vi "Open Item.vi"(8 "error in (no error)":errorcluster, 10 "Item name":string, 11 "Measure Object in":refnum<class "da Base.lvclass">) -> (0 "error out":errorcluster, 3 "Measure Object out":refnum<class "da Base.lvclass">)   [LabVIEW 2016, in "da Base.lvclass"]
uses:
  da Base.lvclass
  C:/Program Files/National Instruments/LabVIEW 2016/vi.lib/ActorFramework/Actor/Actor.lvclass
  <vilib>/ActorFramework/Actor/Actor.lvclass/Actor.ctl
  Da Base Messages/Open Item Msg/Open Item Msg.lvclass/Open Item Msg.ctl
  <vilib>/ActorFramework/Message Enqueuer/Message Enqueuer.lvclass/Message Enqueuer.ctl
  <vilib>/ActorFramework/Message Enqueuer/Enqueue.vi
  Da Base Messages/Open Item Msg/Open Item Msg.lvclass
  C:/Program Files/National Instruments/LabVIEW 2016/vi.lib/ActorFramework/Message/Message.lvclass
  Da Base Messages/Open Front Panel Msg/Open Front Panel Msg.lvclass
  <vilib>/ActorFramework/Message Priority Queue/Priority Enqueue.vi
  <vilib>/ActorFramework/Message Enqueuer/Message Enqueuer.lvclass
  <vilib>/ActorFramework/Actor/Actor.lvclass
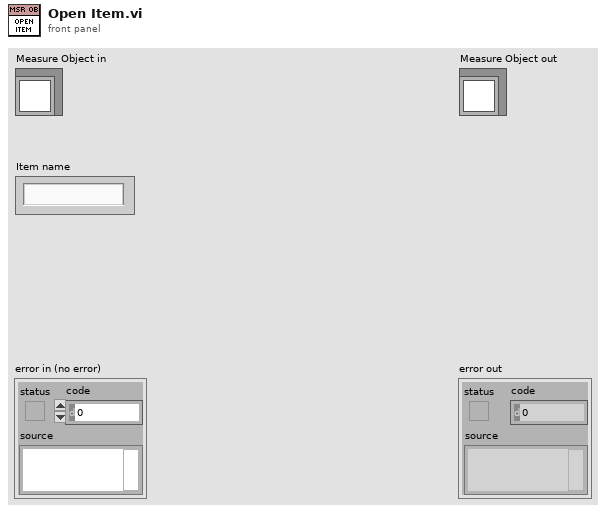
[diagram p1: front panel]
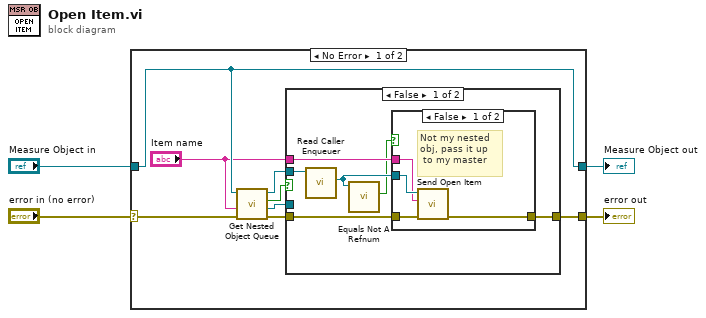
[diagram p0: block diagram]
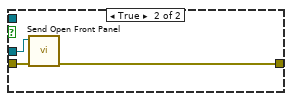
[diagram p3: hidden frame]
diagram:
  n1 = case shown="No Error" "error in (no error)" {
    selector: "error in (no error)" -> [w8 w28]
    tunnel: [w5 w28] -> w3
    tunnel: [w12 w27] -> w1
    tunnel: "Measure Object in" -> [w12 w27]
    frame No Error {
      n2 = call-dynamic "Get Nested Object Queue.vi"("error in (no error)"=w8, "Name"="Item name", "Measure Object in"=w12) -> ("error out"=w6:errorcluster, "Object Enqueuer"=w9:refnum<class "Message Enqueuer.lvclass">, "Found?"=w11:bool, "Measure Object out"=w10:refnum<class "da Base.lvclass">)  [unwired: 5 in]
      n3 = case shown="False" w11 {
        tunnel: w10 -> [w18 _]
        tunnel: w9 -> [_ w26]
        tunnel: "Item name" -> [w17 _]
        tunnel: w6 -> [w16 w25]
        tunnel: [w15 w24] -> w5
        frame False {
          n4 = call <vilib>:"Read Caller Enqueuer.vi"("Actor"=w18) -> ("Caller Enqueuer"=w14:refnum<class "Message Enqueuer.lvclass">)  [unwired: 10 in]
          n5 = call <vilib>:"Equals Not A Refnum.vi"("Message Enqueuer"=w14) -> ("Not a refnum?"=w13:bool)  [unwired: 10 in]
          n6 = case shown="False" w13 {
            tunnel: w14 -> [w22 _]
            tunnel: w17 -> [w21 _]
            tunnel: w16 -> [w20 w23]
            tunnel: [w19 w23] -> w15
            frame False {
              # "Not my nested \nobj, pass it up\n to my master"
              n7 = call "Send Open Item.vi"("error in (no error)"=w20, "Item name"=w21, "Message Enqueuer"=w22) -> ("error out"=w19:errorcluster)  [unwired: 7 in, 1 out]
            }
            frame True {
            }
          }
        }
        frame True {
          n8 = call "Send Open Front Panel.vi"("error in (no error)"=w25, "Message Enqueuer"=w26) -> ("error out"=w24:errorcluster)  [unwired: 8 in, 1 out]
        }
      }
    }
    frame Error {
    }
  }
  "error out" <- w3
  "Measure Object out" <- w1
